vi "Set Start Node.vi"(0 "FSM.Graph In":refnum<class "FSM.Graph.lvclass">, 7 "Index":i32) -> (4 "FSM.Graph Out":refnum<class "FSM.Graph.lvclass">)   [LabVIEW 2020, in "FSM.Graph.lvclass"]
uses:
  FSM.Graph.lvclass
  FSM.Graph.lvclass/FSM.Graph.ctl
  FSM.Node/FSM.Node.lvclass/FSM.Node.ctl
  FSM.Node/Shape.ctl
  FSM.Node/Write Shape.vi
  FSM.Node/Read Shape.vi
  FSM.Node/FSM.Node.lvclass
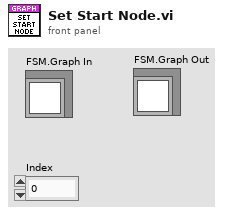
[diagram p1: front panel]
types:
  T1 = typedef "FSM.Node.lvclass/Shape.ctl" = enum16{"Default", "Start", "Action", "End"}
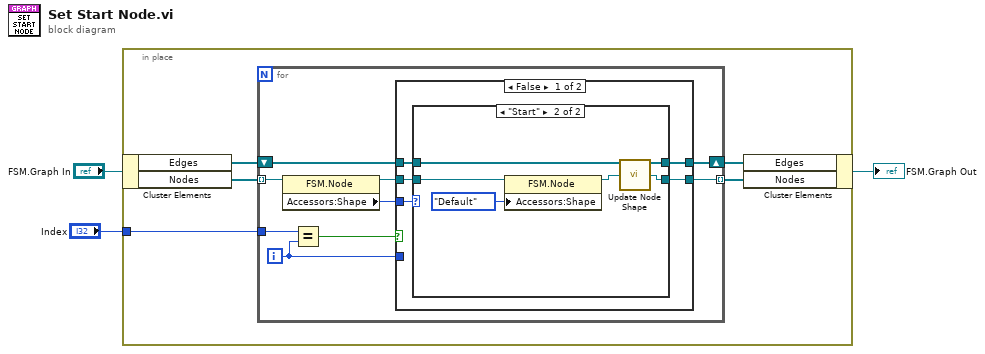
[diagram p0: block diagram]
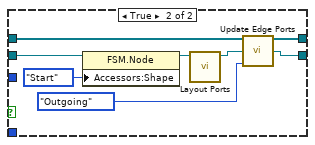
[diagram p3: hidden frame]
diagram:
  n1 = in-place {
    in-place-border: "Index" -> [w7]
    n2 = in-place-cluster #1("FSM.Graph In") -> ("Edges"=w6:refnum<class "FSM.Edge.lvclass">[], "Nodes"=w8:refnum<class "FSM.Node.lvclass">[])
    n3 = for {
      tunnel: w8 -> [w16] mode=indexing
      tunnel: w7 -> [w17]
      tunnel: [w14] -> w4 mode=indexing
      shift-right: [w10] -> w5
      shift-left: w6 -> [w11]
      i -> [w9]
      n4 = property class="FSM.Node"(reference=w16) -> (reference out=w13:refnum<class "FSM.Node.lvclass">, "Accessors:Shape"=w12:T1)  [unwired: 1 in, 1 out]
      n5 = Equal?(x=w17, y=w9) -> (x = y?=w15:bool)
      n6 = case shown="False" w15 {
        tunnel: w13 -> [w20 w38]
        tunnel: [w21 w31] -> w14
        tunnel: w12 -> [w22 _]
        tunnel: w11 -> [w19 w34]
        tunnel: [w18 w35] -> w10
        tunnel: w9 -> [_ _]
        frame False {
          n7 = case shown="\"Start\"" w22 {
            tunnel: [w23 w28] -> w21
            tunnel: w20 -> [w23 w27]
            tunnel: w19 -> [w24 w29]
            tunnel: [w24 w30] -> w18
            frame "Default", Default {
            }
            frame "Start" {
              n8 = property class="FSM.Node"(reference=w27, "Accessors:Shape"=Shape."Default" ("Shape")) -> (reference out=w26:refnum<class "FSM.Node.lvclass">)  [unwired: 1 in, 1 out]
              n9 = call "Update Node Shape.vi"("Edges"=w29, "FSM.Node in"=w26) -> ("Edges Out"=w30:refnum<class "FSM.Edge.lvclass">[], "FSM.Node out"=w28:refnum<class "FSM.Node.lvclass">)  [unwired: 12 in]
            }
          }
        }
        frame True {
          n10 = property class="FSM.Node"(reference=w38, "Accessors:Shape"=Shape."Start" ("Shape")) -> (reference out=w36:refnum<class "FSM.Node.lvclass">)  [unwired: 1 in, 1 out]
          n11 = call "Layout Ports.vi"("Node in"=w36) -> ("Node out"=w33:refnum<class "FSM.Node.lvclass">)  [unwired: 9 in, 1 out]
          n12 = call "Update Edge Ports.vi"("Edges In"=w34, "FSM.Node In"=w33, "Edges"=enum16{"Incoming", "Outgoing"}."Outgoing") -> ("Edges Out"=w35:refnum<class "FSM.Edge.lvclass">[], "FSM.Node thru"=w31:refnum<class "FSM.Node.lvclass">)  [unwired: 11 in]
        }
      }
    }
    n13 = in-place-cluster #1("Edges"=w5, "Nodes"=w4) -> (→"FSM.Graph Out":refnum<class "FSM.Graph.lvclass">)
  }
